vi "LocalGoal_Msg.vi"(8 "error in (no error)":errorcluster caption="错误输入（无错误）", 10 "值(信号)":T1, 11 "RemoteP3AT输入":refnum<class "RemoteP3AT.lvclass">) -> (0 "error out":errorcluster caption="错误输出", 3 "RemoteP3AT输出":refnum<class "RemoteP3AT.lvclass">)   [LabVIEW 2014, in "RemoteP3AT.lvlib" / "RemoteP3AT.lvclass"]
uses:
  RemoteP3AT.lvclass
  ctl/Point.ctl
  RemoteP3AT.lvclass/RemoteP3AT.ctl
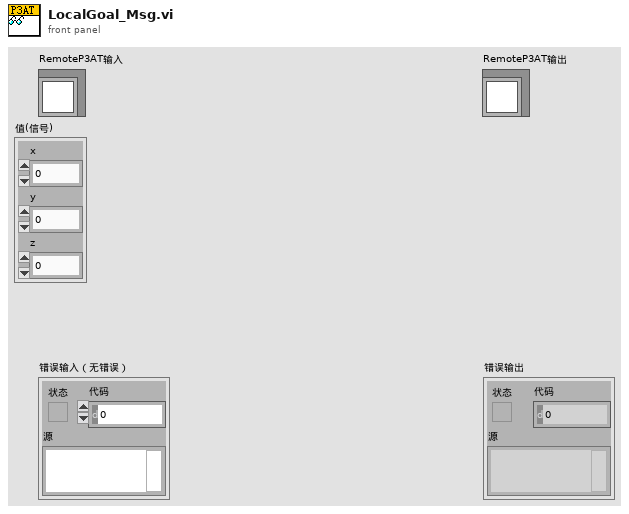
[diagram p1: front panel]
types:
  T1 = typedef "Point.ctl" = cluster{"x":dbl, "y":dbl, "z":dbl}
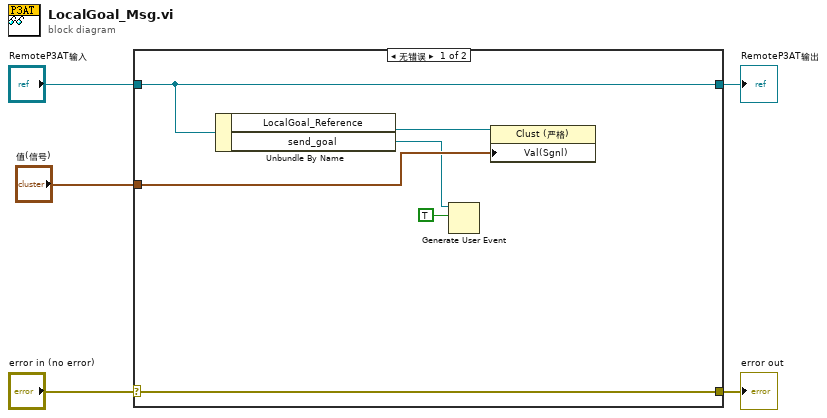
[diagram p0: block diagram]
diagram:
  n1 = case shown="无错误" "error in (no error)" {
    selector: "error in (no error)" -> [w11 w12]
    tunnel: [w11 w12] -> w4
    tunnel: [w10 w13] -> w2
    tunnel: "RemoteP3AT输入" -> [w10 w13]
    tunnel: "值(信号)" -> [w8 _]
    frame No Error {
      n2 = Unbundle By Name(w10) -> ("LocalGoal_Reference"=w9:refnum<vi>, "send_goal"=w6:refnum<user-event>)
      n3 = Generate User Event(user event=w6, event data cluster=TRUE ("event data")) -> ()  [unwired: 2 in, 2 out]
      n4 = property class="Clust (严格)"(reference=w9, "Val(Sgnl)"=w8) -> ()  [unwired: 1 in, 2 out]
    }
    frame Error {
    }
  }
  "error out" <- w4
  "RemoteP3AT输出" <- w2
